vi "pid pwm custom.vi"() -> ()   [LabVIEW 2012]
doc: "This VI is an example of using the PID VI for a PWM application. For a real application all that is needed is the PID VI and the Output to PWM Logic. Together these can be put in the while loop of a real application.\n\nThis example has defaults tuned to the plant."
uses:
  <vilib>/addons/control/pid/pid.llb/PID (DBL).vi
  <vilib>/addons/control/pid/NI_PID_pid.lvlib
panel:
  in  "PID gains":T1={"proportional gain (Kc)"=0.001, "integral time (Ti, min)"=30.0, "derivative time (Td, min)"=0.0} {"derivative time (Td, min)" format="%.3f"; "integral time (Ti, min)" format="%.3f"; "proportional gain (Kc)" format="%.3f"}
  out "PWM Output":bool
  out "Waveform Chart":dbl[][](graph)
  in  "stop":bool
  in  "Start process variable":dbl
  in  "Setpoint":dbl=500.0 format="%.2f"
  # "Overview: This VI is an example of using the PID VI for a PWM application. For a real application all that is needed is the PID VI and the Output to PWM Logic. Together these can be put in the while loop of a real application.\nRequirements: NI LabVIEW Professional Development System 2012 or compatible, PID and Fuzzy Logic Toolkit 2012 or compatible.\nInstructions: \n1. Set the Setpoint and Start Process Variable.\n2. Configure the PID gains.\n3. Run the VI."
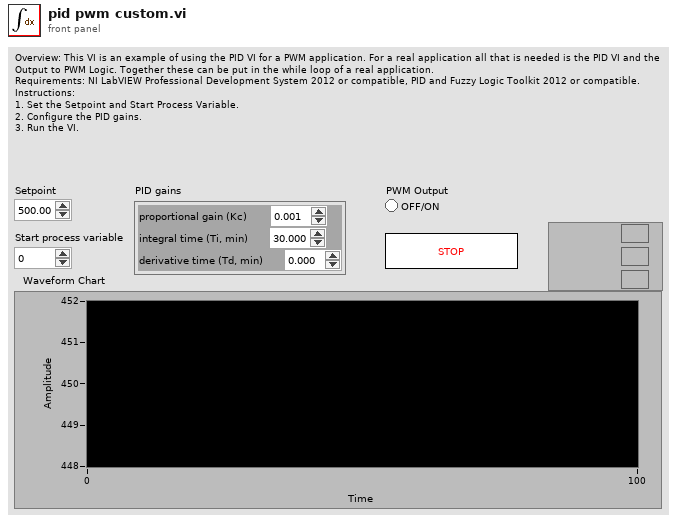
[diagram p1: front panel]
types:
  T1 = cluster{"proportional gain (Kc)":dbl, "integral time (Ti, min)":dbl, "derivative time (Td, min)":dbl}
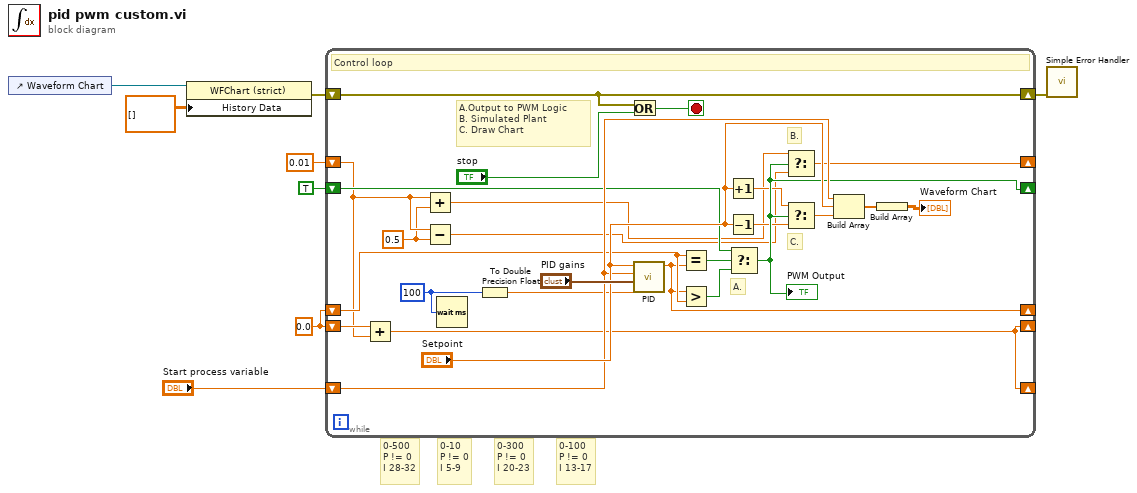
[diagram p0: block diagram]
diagram:
  w6 = 0.0 ("output")
  # "0-100\nP != 0\nI 13-17"
  # "0-300\nP != 0\nI 20-23"
  # "0-10\nP != 0\nI 5-9"
  # "0-500\nP != 0\nI 28-32"
  n1 = control-ref of="Waveform Chart"() -> (w4:refnum<vi>)
  n2 = property class="WFChart (strict)"(reference=w4, "History Data"=dbl[][] []) -> (error out=w3:errorcluster)  [unwired: 1 in, 1 out]
  n3 = while {
    shift-right: [w24] -> _
    shift-left: "Start process variable" -> [w30]
    shift-right: [w28] -> _
    shift-left: w6 -> [w29]
    shift-right: [w26] -> _
    shift-left: TRUE -> [w27]
    shift-right: [w24] -> _
    shift-left: w6 -> [w25]
    shift-right: [w22] -> _
    shift-left: 0.01 -> [w23]
    shift-right: [w19] -> w2
    shift-left: w3 -> [w19]
    stop <- w20 stop-if-true
    w11 = 0.5 ("x")
    w32 = u32 100 ("milliseconds to wait")
    # "B."
    # "C."
    # "A."
    # "A.Output to PWM Logic \nB. Simulated Plant\nC. Draw Chart"
    # "Control loop"
    n4 = Add(x=w25, y=w23) -> (x+y=w24:dbl)
    n5 = Add(x=w23, y=w11) -> (x+y=w12:dbl)
    n6 = Subtract(x=w23, y=w11) -> (x-y=w10:dbl)
    n7 = Wait (ms)(milliseconds to wait=w32) -> ()  [unwired: 1 out]
    n8 = To Double Precision Float(number=w32) -> (double precision float=w9:dbl)
    n9 = Or(x=w19, y="stop") -> (x .or. y?=w20:bool)
    n10 = call-poly <vilib>:"PID.vi"("dt (s)"=w9, "PID gains"="PID gains", "process variable"=w30, "setpoint"="Setpoint") -> ("output"=w28:dbl)  [unwired: 6 in, 1 out]
    n11 = Equal?(x=w29, y=w28) -> (x = y?=w18:bool)
    n12 = Greater?(x=w28, y=w29) -> (0:w17:bool)
    n13 = Increment(x="Setpoint") -> (x+1=w16:dbl)
    n14 = Decrement(x="Setpoint") -> (x-1=w15:dbl)
    n15 = Select(t=w27, s=w18, f=w17) -> (s? t:f=w26:bool)
    "PWM Output" <- w26
    n16 = Select(t=w12, s=w26, f=w10) -> (s? t:f=w22:dbl)
    n17 = Select(t=w16, s=w26, f=w15) -> (s? t:f=w14:dbl)
    n18 = Build Array(w30, "Setpoint", w14) -> (w13:dbl[])
    n19 = Build Array(w13) -> (→"Waveform Chart":dbl[][])
  }
  n20 = call <vilib>:"Simple Error Handler.vi"("error in (no error)"=w2) -> ()  [unwired: 4 in, 5 out]
